vi "Joystick interpolation Full.vi"() -> ()   [LabVIEW 2017]
uses:
  <vilib>/Analysis/1siggen.llb/Ramp Pattern by Delta.vi
  <vilib>/gmath/NI_Gmath.lvlib
  <vilib>/Analysis/NI_AALBase.lvlib
panel:
  in  "Numeric":dbl=1000.0 format="%#_13g"
  in  "method":i32(ring)=3 items=["nearest", "linear", "spline", "cubic Hermite", "Lagrange"]
  in  "Slide 5":dbl(slide) scale=0.0..1.0
  in  "Slide 6":dbl(slide) scale=0.0..1.0
  out "Power":dbl(slide) scale=-1.0..1.0
  in  "Joystick Sim":dbl(slide) scale=-1.0..1.0
  in  "Slide 4":dbl(slide) scale=0.0..1.0
  in  "Slide 3":dbl(slide) scale=0.0..1.0
  in  "Slide 2":dbl(slide) scale=0.0..1.0
  in  "Slide":dbl(slide) scale=0.0..1.0
  out "Interpolated Data":dbl[][](array[numeric])
  out "1D Interpolation Graph":cluster{"yi":dbl[], "ramp data":dbl[]}[](graph)
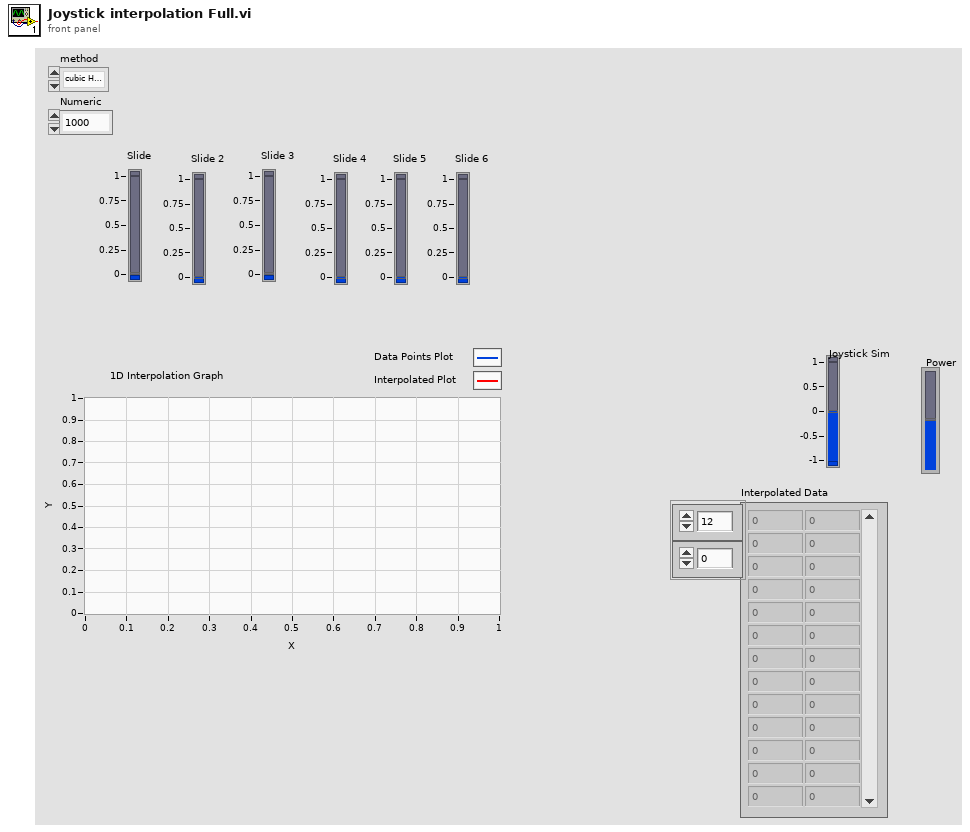
[diagram p1: front panel]
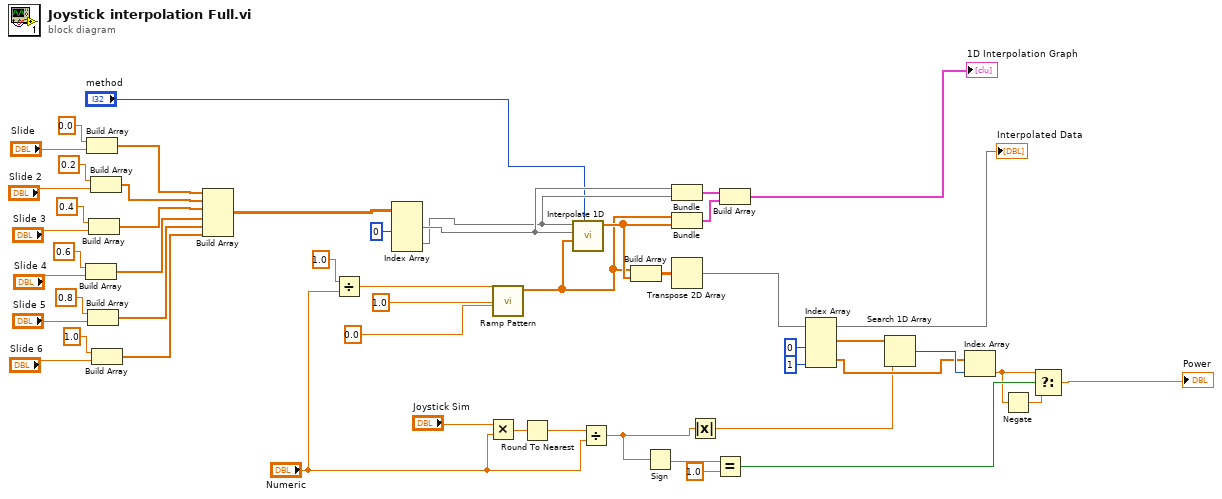
[diagram p0: block diagram]
diagram:
  n1 = Build Array(0.6 ("element"), "Slide 4") -> (w40:dbl[])
  n2 = Build Array(0.0 ("element"), "Slide") -> (w43:dbl[])
  n3 = Build Array(0.8 ("element"), "Slide 5") -> (w30:dbl[])
  n4 = Build Array(0.4 ("element"), "Slide 3") -> (w41:dbl[])
  n5 = Build Array(0.2 ("element"), "Slide 2") -> (w42:dbl[])
  n6 = Build Array(1.0 ("element"), "Slide 6") -> (w29:dbl[])
  n7 = Build Array(w43, w42, w41, w40, w30, w29) -> (w7:dbl[][])
  n8 = Divide(x=1.0 ("delta"), y="Numeric") -> (x/y=w2:dbl)
  n9 = Index Array(array=w7, index (col) #1=0 ("disabled index (col)")) -> (element #1=w15:dbl[], element #2=w14:dbl[])  [unwired: 3 in]
  n10 = Multiply(x="Joystick Sim", y="Numeric") -> (x*y=w27:dbl)
  n11 = call-poly <vilib>:"Ramp Pattern.vi"("start"=0.0, "end"=1.0, "delta"=w2) -> ("Ramp Pattern"=w11:dbl[])  [unwired: 6 in, 2 out]
  n12 = Round To Nearest(number=w27) -> (nearest integer value=w26:dbl)
  n13 = call <vilib>:"Interpolate 1D.vi"("method"="method", "xi"=w11, "X"=w15, "Y"=w14) -> ("yi"=w12:dbl[])  [unwired: 5 in, 2 out]
  n14 = Divide(x=w26, y="Numeric") -> (x/y=w25:dbl)
  n15 = Build Array(w11, w12) -> (w13:dbl[][])
  n16 = Sign(1:w25) -> (0:w23:dbl)
  n17 = Bundle(w15, w14) -> (w16:cluster{dbl[], dbl[]})  [unwired: 1 in]
  n18 = Bundle("Ramp Pattern"=w11, "yi"=w12) -> (w17:cluster{"Ramp Pattern":dbl[], "yi":dbl[]})  [unwired: 1 in]
  n19 = Transpose 2D Array(2D array=w13) -> (transposed array=w5:dbl[][])
  "Interpolated Data" <- w5
  n20 = Absolute Value(x=w25) -> (abs(x)=w24:dbl)
  n21 = Equal?(x=w23, y=1.0) -> (x = y?=w21:bool)
  n22 = Build Array(w16, w17) -> (→"1D Interpolation Graph":cluster{"Ramp Pattern":dbl[], "yi":dbl[]}[])
  n23 = Index Array(array=w5, index (col) #1=0 ("disabled index (col)"), index (col) #2=1 ("index (col)")) -> (element #1=w35:dbl[], element #2=w36:dbl[])  [unwired: 2 in]
  n24 = Search 1D Array(1D array=w35, element=w24) -> (index of element=w39:i32)  [unwired: 1 in]
  n25 = Index Array(array=w36, index=w39) -> (element=w19:dbl)
  n26 = Negate(x=w19) -> (-x=w20:dbl)
  n27 = Select(t=w19, s=w21, f=w20) -> (s? t:f=→"Power":dbl)
